vi "upper bound check.vi"(8 "error in (no error)":errorcluster, 10 "pointer to shared memory":u64, 11 "upper bound (inclusive)":u64) -> (0 "error out":errorcluster)   [LabVIEW 2018, in "linuxSharedMemory.lvlib"]
uses:
  linuxSharedMemory.lvlib
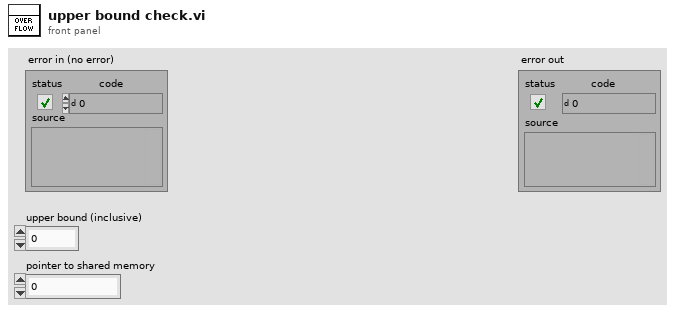
[diagram p1: front panel]
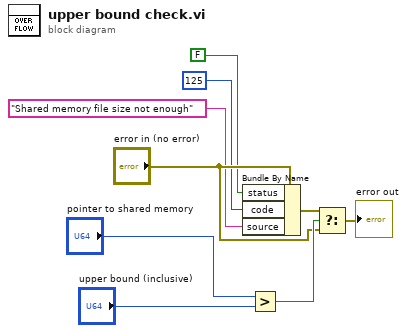
[diagram p0: block diagram]
diagram:
  n1 = Bundle By Name(cluster="error in (no error)", "status"=FALSE, "code"=125, "source"="Shared memory file size not enough") -> (w6:errorcluster)
  n2 = Greater?(x="pointer to shared memory", y="upper bound (inclusive)") -> (0:w9:bool)
  n3 = Select(t=w6, s=w9, f="error in (no error)") -> (s? t:f=→"error out":errorcluster)
